vi "Set Read Filter.vi"(8 "error in (no error)":errorcluster, 10 "PCAP Filter Exp":string, 11 "pcap reference in":u64) -> (0 "error out":errorcluster, 3 "pcap reference out":u64)   [LabVIEW 2025, in "Automotive Ethernet Bus Monitor UI.lvlib" / "lvwpcap.lvlib"]
uses:
  lvwpcap.lvlib
  lvwpcap.dll
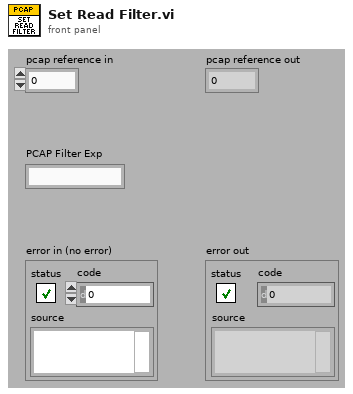
[diagram p1: front panel]
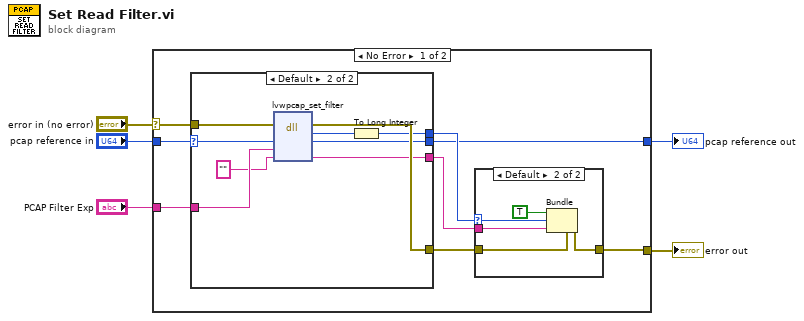
[diagram p0: block diagram]
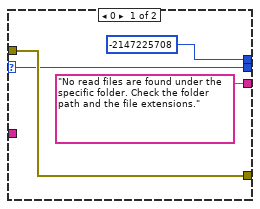
[diagram p2: hidden frame]
diagram:
  n1 = case shown="No Error" "error in (no error)" {
    selector: "error in (no error)" -> [w12 w34]
    tunnel: [w10 w34] -> w5
    tunnel: [w9 w33] -> w3
    tunnel: "pcap reference in" -> [w6 w33]
    tunnel: "PCAP Filter Exp" -> [w7 _]
    frame No Error {
      n2 = case shown="Default" w6 {
        selector: w6 -> [w15 w19]
        tunnel: [-2147225708 ("return type") w18] -> w13
        tunnel: w12 -> [w17 w25]
        tunnel: [w17 w24] -> w11
        tunnel: [w15 w23] -> w9
        tunnel: ["No read files are found under the specific folder. Check the folder path and the file extensions." ("error_string") w22] -> w8
        tunnel: w7 -> [_ w21]
        frame 0 {
        }
        frame Default {
          n3 = dll-call lib="lvwpcap.dll" fn="lvwpcap_set_filter"(error in=w25, "pcap"=w19, "pcap_filter"=w21, "error_string"="") -> (error out=w24:errorcluster, "return type"=w26:u64, "pcap"=w23:u64, "error_string"=w22:string)  [unwired: 3 in, 1 out]
          n4 = To Long Integer(number=w26) -> (32bit integer=w18:i32)
        }
      }
      n5 = case shown="Default" w13 {
        selector: w13 -> [_ w31]
        tunnel: w8 -> [_ w30]
        tunnel: w11 -> [w27 w32]
        tunnel: [w27 w28] -> w10
        frame 0 {
        }
        frame Default {
          n6 = Bundle(cluster=w32, "status"=TRUE, "code"=w31, "source"=w30) -> (w28:errorcluster)
        }
      }
    }
    frame Error {
    }
  }
  "error out" <- w5
  "pcap reference out" <- w3
